vi "Read Environment Variable.vi"() -> ()   [LabVIEW 2021, in "NI Measurement Plug-In SDK.lvlib"]
uses:
  NI Measurement Plug-In SDK.lvlib
panel:
  in  "Env Variable":string="NIDISCOVERY_CLUSTERID"
  out "Environment Variable Value":string
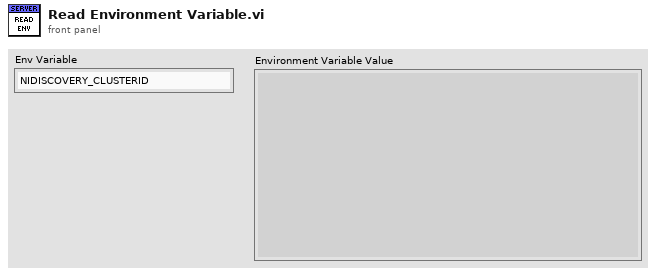
[diagram p1: front panel]
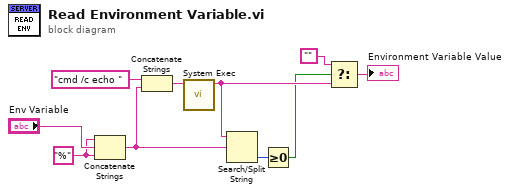
[diagram p0: block diagram]
diagram:
  w2 = "%" ("command line")
  n1 = Concatenate Strings(w2, "Env Variable", w2) -> (w1:string)
  n2 = Concatenate Strings("cmd /c echo " ("command line"), w1) -> (w9:string)
  n3 = call <vilib>:"System Exec.vi"("command line"=w9) -> ("standard output"=w6:string)  [unwired: 7 in, 3 out]
  n4 = Search/Split String(string=w6, search string/char (-)=w1) -> (offset of match=w5:i32)  [unwired: 1 in, 2 out]
  n5 = Greater Or Equal To 0?(x=w5) -> (x >= 0?=w4:bool)
  n6 = Select(t="", s=w4, f=w6) -> (s? t:f=→"Environment Variable Value":string)
